vi "Write Core.vi"(8 "error in":errorcluster, 9 "Timeout (1s)":dbl[unit]=1.0, 10 "PV":refnum<class "PV.lvclass">, 11 "BNT_SLTagConnection in":refnum<class "BNT_SLTagConnection.lvclass">) -> (0 "error out":errorcluster, 1 "timed out":bool, 3 "BNT_SLTagConnection out":refnum<class "BNT_SLTagConnection.lvclass">)   [LabVIEW 2019, in "BNT_SLTagConnection.lvlib" / "BNT_SLTagConnection.lvclass"]
doc: "Publish a process variable."
uses:
  BNT_SLTagConnection.lvclass
  C:/Users/Holger/Documents/LVP/CSPP/CSPP-Template/Packages/CSPP_Core/Classes/CSPP_ProcessVariables/PVConnection/PVConnection.lvclass
  C:/Users/Holger/Documents/LVP/CSPP/CSPP-Template/Packages/CSPP_Core/Classes/CSPP_BaseClasses/Base/CSPP_Base.lvclass
  CSPP_Core/Classes/CSPP_ProcessVariables/ProcessVariable/PV.lvclass
  BNT_SLTagConnection.lvclass/BNT_SLTagConnection.ctl
  <vilib>/Skyline/Tag/Wrapper/Wrapper_class/NI Skyline Tag.lvclass/NI Skyline Tag.ctl
  CSPP_Core/Classes/CSPP_ProcessVariables/ProcessVariable/PV.lvclass/PV.ctl
  CSPP_Core/Libraries/Base/Severity.ctl
  CSPP_Core/Classes/CSPP_BaseClasses/Base/CSPP_Base.lvclass/CSPP_Base.ctl
  CSPP_Core/Classes/CSPP_ProcessVariables/PVConnection/PVConnection.lvclass/PVConnection.ctl
  CSPP_Core/Classes/CSPP_ProcessVariables/ProcessVariable/Read Data.vi
  CSPP_Core/Classes/CSPP_ProcessVariables/ProcessVariable/Read Timestamp.vi
  <vilib>/Skyline/Tag/Wrapper/Wrapper_class/Read Tag Path.vi
  <vilib>/Skyline/Tag/Wrapper/Wrapper_class/Write Tag (I32).vi
  <vilib>/Skyline/Tag/Wrapper/Wrapper_class/Write Tag (DBL).vi
  <vilib>/Skyline/Tag/Wrapper/Wrapper_class/Write Tag (String).vi
  <vilib>/Skyline/Tag/Wrapper/Wrapper_class/Write Tag (Boolean).vi
  <vilib>/Skyline/Tag/Wrapper/Wrapper_class/Write Tag (U64).vi
  <vilib>/Skyline/Tag/Wrapper/Wrapper_class/Write Tag (Timestamp).vi
  <vilib>/Skyline/Tag/Wrapper/Wrapper_class/NI Skyline Tag.lvclass
  CSPP_Core/Libraries/Utilities/CSPP_Utilities.lvlib
  CSPP_Core/Classes/CSPP_ProcessVariables/PVConnection/PVConnection.lvclass
  CSPP_Core/Classes/CSPP_BaseClasses/Base/CSPP_Base.lvclass
  CSPP_Core/Libraries/Base/CSPP_Base.lvlib
  BNT_SLTools.lvlib
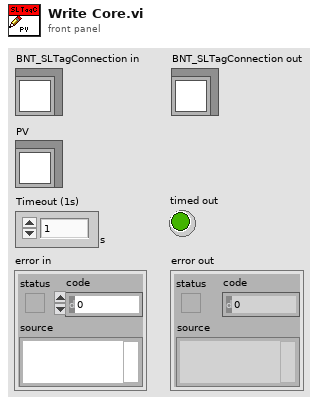
[diagram p1: front panel]
types:
  T1 = cluster{"Read Access":enum8{"Allowed", "Required", "None"}, "Write Access":enum8{"Allowed", "Required", "None"}}
  T2 = typedef "CSPP_Base.lvlib/Severity.ctl" = enum16{"emergency", "alert", "critical", "error", "warning", "notice", "info", "debug"}
  T3 = typedef "NI Skyline Tag.lvlib/DataType.ctl" = enum32{"Double", "I32", "String", "Boolean", "U64", "Timestamp"}
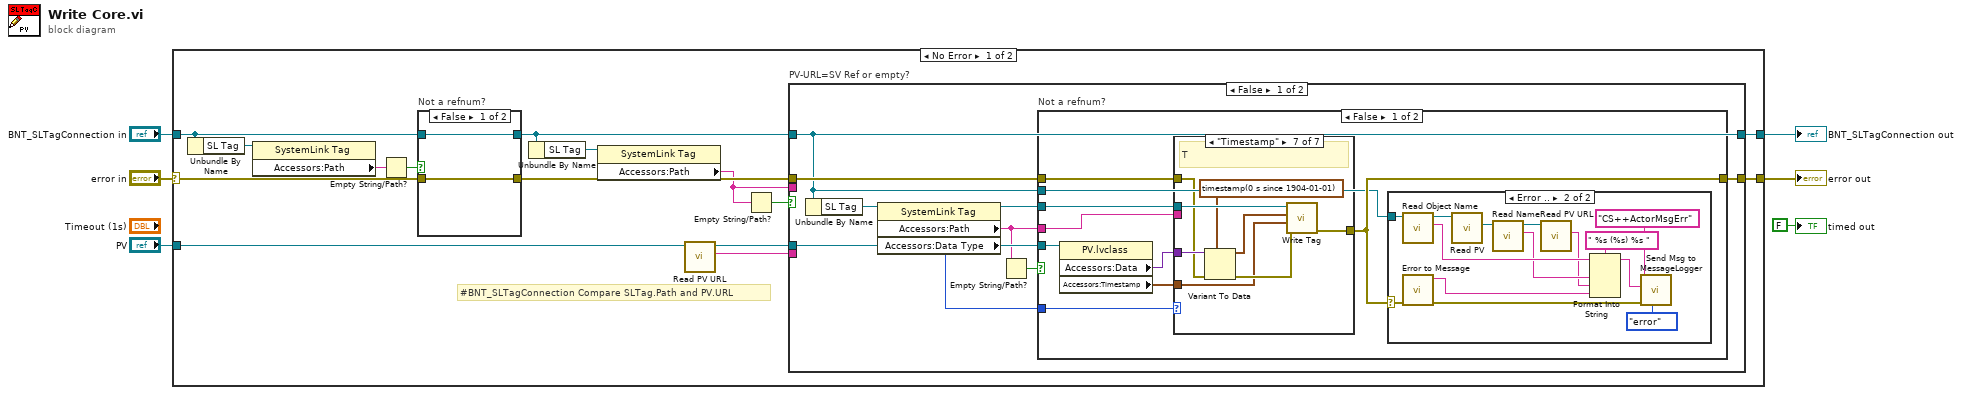
[diagram p0: block diagram]
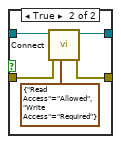
[diagram p2: hidden frame]
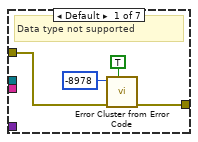
[diagram p3: hidden frame]
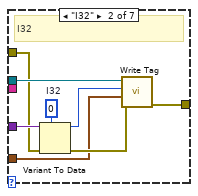
[diagram p4: hidden frame]
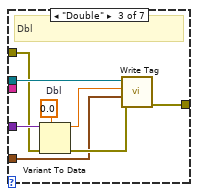
[diagram p5: hidden frame]
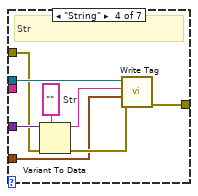
[diagram p6: hidden frame]
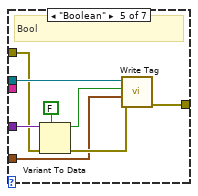
[diagram p7: hidden frame]
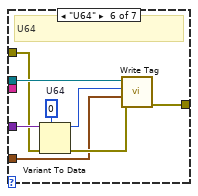
[diagram p8: hidden frame]
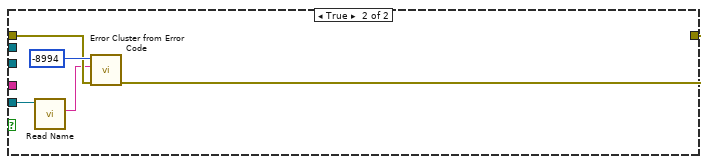
[diagram p10: hidden frame]
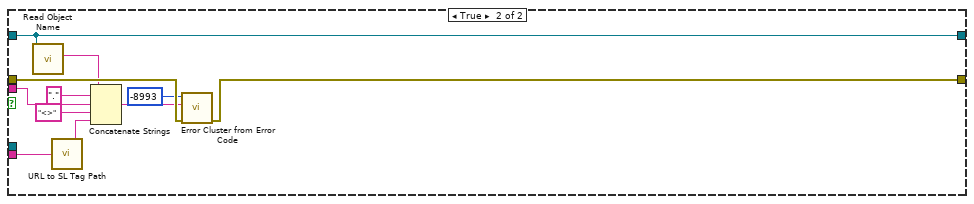
[diagram p11: hidden frame]
diagram:
  n1 = case shown="No Error" "error in" {
    selector: "error in" -> [w15 w130]
    tunnel: [w21 w130] -> w6
    tunnel: [w20 w129] -> w5
    tunnel: "PV" -> [w19 _]
    tunnel: "BNT_SLTagConnection in" -> [w14 w129]
    frame No Error {
      # "#BNT_SLTagConnection Compare SLTag.Path and PV.URL"
      n2 = Unbundle By Name(w14) -> ("SL Tag"=w12:refnum<class "NI Skyline Tag.lvclass">)
      n3 = property class="SystemLink Tag"(reference=w12) -> ("Accessors:Path"=w11:string)  [unwired: 1 in, 2 out]
      n4 = Empty String/Path?(string/path=w11) -> (empty?=w17:bool)
      n5 = case "Not a refnum?" shown="False" w17 {
        tunnel: w14 -> [w22 w28]
        tunnel: [w22 w27] -> w13
        tunnel: w15 -> [w23 w26]
        tunnel: [w23 w25] -> w16
        frame False {
        }
        frame True {
          n6 = call "Connect.vi"("Access (R/W allowed)"=T1 {"Read Access"=enum."Allowed", "Write Access"=enum."Required"}, "Error In"=w26, "PVConnection in"=w28) -> ("Error Out"=w25:errorcluster, "PVConnection out"=w27:refnum<class "BNT_SLTagConnection.lvclass">)  [unwired: 7 in]
        }
      }
      n7 = Unbundle By Name(w13) -> ("SL Tag"=w10:refnum<class "NI Skyline Tag.lvclass">)
      n8 = property class="SystemLink Tag"(reference=w10) -> ("Accessors:Path"=w8:string)  [unwired: 1 in, 2 out]
      n9 = call "Read PV URL.vi"("PV in"=w19) -> ("PV URL"=w7:string, "PV out"=w18:refnum<class "PV.lvclass">)  [unwired: 8 in, 1 out]
      n10 = Empty String/Path?(string/path=w8) -> (empty?=w9:bool)
      n11 = case "PV-URL=SV Ref or empty?" shown="False" w9 {
        tunnel: [w36 w127] -> w21
        tunnel: [w33 w121] -> w20
        tunnel: w13 -> [w33 w121]
        tunnel: w16 -> [w37 w128]
        tunnel: w18 -> [w35 _]
        tunnel: w8 -> [_ w125]
        tunnel: w7 -> [_ w119]
        frame False {
          n12 = Unbundle By Name(w33) -> ("SL Tag"=w32:refnum<class "NI Skyline Tag.lvclass">)
          n13 = property class="SystemLink Tag"(reference=w32) -> (reference out=w30:refnum<class "NI Skyline Tag.lvclass">, "Accessors:Path"=w31:string, "Accessors:Data Type"=w29:T3)  [unwired: 1 in, 1 out]
          n14 = Empty String/Path?(string/path=w31) -> (empty?=w34:bool)
          n15 = case "Not a refnum?" shown="False" w34 {
            tunnel: w31 -> [w43 _]
            tunnel: w37 -> [w46 w116]
            tunnel: [w45 w115] -> w36
            tunnel: w35 -> [w40 w114]
            tunnel: w33 -> [w44 _]
            tunnel: w30 -> [w42 _]
            tunnel: w29 -> [w41 _]
            frame False {
              n16 = property class="PV.lvclass"(reference=w40) -> ("Accessors:Data"=w39:variant, "Accessors:Timestamp"=w38:timestamp)  [unwired: 1 in, 2 out]
              n17 = case shown="\"Timestamp\"" w41 {
                tunnel: w46 -> [w47 w54 w62 w70 w78 w86 w94]
                tunnel: [w48 w58 w66 w74 w82 w90 w98] -> w45
                tunnel: w43 -> [_ _ _ _ _ _ _]
                tunnel: w42 -> [_ w57 w65 w73 w81 w89 w97]
                tunnel: w39 -> [_ w56 w64 w72 w80 w88 w96]
                tunnel: w38 -> [_ w51 w59 w67 w75 w83 w92]
                frame Default {
                  # "Data type not supported"
                  n18 = call "Error Cluster from Error Code.vi"("show call chain? (False)"=TRUE, "Error In"=w47, "Error Code (0)"=-8978 ("error code (0)")) -> ("Error Out"=w48:errorcluster)  [unwired: 8 in]
                }
                frame "I32" {
                  w52 = 0  # I32
                  # "I32"
                  n19 = Variant To Data(error in=w54, type=w52, Variant=w56) -> (data=w53:i32, error out=w55:errorcluster)
                  n20 = call-poly <vilib>:"Write Tag.vi"("error in (no error)"=w55, "time stamp"=w51, "value"=w53, "tag in"=w57) -> ("error out"=w58:errorcluster)  [unwired: 6 in, 1 out]
                }
                frame "Double" {
                  w60 = 0.0  # Dbl
                  # "Dbl"
                  n21 = Variant To Data(error in=w62, type=w60, Variant=w64) -> (data=w61:dbl, error out=w63:errorcluster)
                  n22 = call-poly <vilib>:"Write Tag.vi"("error in (no error)"=w63, "time stamp"=w59, "value"=w61, "tag in"=w65) -> ("error out"=w66:errorcluster)  [unwired: 6 in, 1 out]
                }
                frame "String" {
                  w68 = ""  # Str
                  # "Str"
                  n23 = Variant To Data(error in=w70, type=w68, Variant=w72) -> (data=w69:string, error out=w71:errorcluster)
                  n24 = call-poly <vilib>:"Write Tag.vi"("error in (no error)"=w71, "time stamp"=w67, "value"=w69, "tag in"=w73) -> ("error out"=w74:errorcluster)  [unwired: 6 in, 1 out]
                }
                frame "Boolean" {
                  # "Bool"
                  n25 = Variant To Data(error in=w78, type=FALSE, Variant=w80) -> (data=w77:bool, error out=w79:errorcluster)
                  n26 = call-poly <vilib>:"Write Tag.vi"("error in (no error)"=w79, "time stamp"=w75, "value"=w77, "tag in"=w81) -> ("error out"=w82:errorcluster)  [unwired: 6 in, 1 out]
                }
                frame "U64" {
                  w84 = u64 0  # U64
                  # "U64"
                  n27 = Variant To Data(error in=w86, type=w84, Variant=w88) -> (data=w85:u64, error out=w87:errorcluster)
                  n28 = call-poly <vilib>:"Write Tag.vi"("error in (no error)"=w87, "time stamp"=w83, "value"=w85, "tag in"=w89) -> ("error out"=w90:errorcluster)  [unwired: 6 in, 1 out]
                }
                frame "Timestamp" {
                  # "T"
                  n29 = Variant To Data(error in=w94, type=timestamp(0 s since 1904-01-01) ("T"), Variant=w96) -> (data=w93:timestamp, error out=w95:errorcluster)
                  n30 = call-poly <vilib>:"Write Tag.vi"("error in (no error)"=w95, "time stamp"=w92, "value"=w93, "tag in"=w97) -> ("error out"=w98:errorcluster)  [unwired: 6 in, 1 out]
                }
              }
              n31 = case shown="Error .." w45 {
                selector: w45 -> [_ w100]
                tunnel: w44 -> [_ w99]
                frame No Error {
                }
                frame Error {
                  n32 = call "Read Object Name.vi"("Base in"=w99) -> ("Object Name"=w107:string, "Base out"=w106:refnum<class "BNT_SLTagConnection.lvclass">)  [unwired: 8 in, 1 out]
                  n33 = call "Error to Message.vi"("Error In"=w100) -> ("Error Out"=w109:errorcluster, "Error Message"=w110:string)  [unwired: 9 in]
                  n34 = call "Read PV.vi"("PVConnection in"=w106) -> ("PV"=w105:refnum<class "PV.lvclass">)  [unwired: 8 in, 2 out]
                  n35 = call "Read Name.vi"("PV in"=w105) -> ("Name"=w103:string, "PV out"=w104:refnum<class "PV.lvclass">)  [unwired: 8 in, 1 out]
                  n36 = call "Read PV URL.vi"("PV in"=w104) -> ("PV URL"=w102:string)  [unwired: 8 in, 2 out]
                  n37 = Format Into String(format string=" %s (%s) %s ", initial string=w107, w103, w102, w110) -> (resulting string=w112:string)  [unwired: 1 in, 1 out]
                  n38 = call "Send Msg to MessageLogger.vi"("Severity Code (info)"=Severity."error", "Error In"=w109, "Message Content"=w112, "Message Tag"="CS++ActorMsgErr") -> ()  [unwired: 7 in, 1 out]
                }
              }
            }
            frame True {
              n39 = call "Read Name.vi"("PV in"=w114) -> ("Name"=w113:string)  [unwired: 8 in, 2 out]
              n40 = call "Error Cluster from Error Code.vi"("Error In"=w116, "Error Message (\"\")"=w113, "Error Code (0)"=-8994 ("error code (0)")) -> ("Error Out"=w115:errorcluster)  [unwired: 8 in]
            }
          }
        }
        frame True {
          n41 = call "Read Object Name.vi"("Base in"=w121) -> ("Object Name"=w120:string)  [unwired: 8 in, 2 out]
          n42 = call "URL to SL Tag Path.vi"("URL"=w119) -> ("SL Tag Path"=w118:string)
          n43 = Concatenate Strings(w120, "." ("string"), w125, "<>" ("string"), w118) -> (w123:string)
          n44 = call "Error Cluster from Error Code.vi"("Error In"=w128, "Error Message (\"\")"=w123, "Error Code (0)"=-8993 ("error code (0)")) -> ("Error Out"=w127:errorcluster)  [unwired: 8 in]
        }
      }
    }
    frame Error {
    }
  }
  "error out" <- w6
  "BNT_SLTagConnection out" <- w5
  "timed out" <- FALSE ("timed out")
